vi "Default8bitColourMap.vi"() -> (0 "Default 8-bit Colour Map":u32[](array[numeric]))   [LabVIEW 2020, in "g_ar_toolkit.image.lvlib"]
uses:
  g_ar_toolkit.image.lvlib
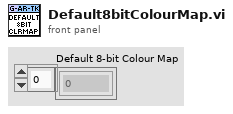
[diagram p1: front panel]
types:
  T1 = cluster{"left":i16, "top":i16, "right":i16, "bottom":i16}
  T2 = typedef "imagedata.ctl" = cluster{"image type":i32, "image depth":i32, "image":u8[], "mask":u8[], "colors":u32[], "Rectangle":cluster{"left":i16, "top":i16, "right":i16, "bottom":i16}}
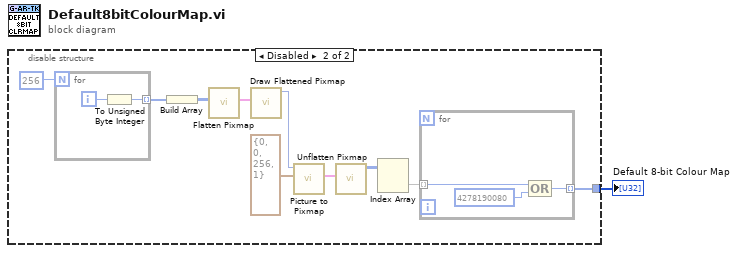
[diagram p0: block diagram]
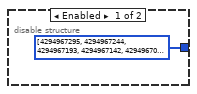
[diagram p2: hidden frame]
diagram:
  n1 = disable-structure shown="Disabled" {
    disable-tunnel: [u32[] [4294967295, 4294967244, 4294967193, 4294967142, 4294967091, 4294967040, 4294954239, 4294954188, 4294954137, 4294954086, 4294954035, 4294953984, 4294941183, 4294941132, 4294941081, 4294941030, 4294940979, 4294940928, 4294928127, 4294928076, 4294928025, 4294927974, 4294927923, 4294927872, 4294915071, 4294915020, 4294914969, 4294914918, 4294914867, 4294914816, 4294902015, 4294901964, 4294901913, 4294901862, 4294901811, 4294901760, 4291624959, 4291624908, 4291624857, 4291624806, 4291624755, 4291624704, 4291611903, 4291611852, 4291611801, 4291611750, 4291611699, 4291611648, 4291598847, 4291598796, 4291598745, 4291598694, 4291598643, 4291598592, 4291585791, 4291585740, 4291585689, 4291585638, 4291585587, 4291585536, 4291572735, 4291572684, 4291572633, 4291572582, 4291572531, 4291572480, 4291559679, 4291559628, 4291559577, 4291559526, 4291559475, 4291559424, 4288282623, 4288282572, 4288282521, 4288282470, 4288282419, 4288282368, 4288269567, 4288269516, 4288269465, 4288269414, 4288269363, 4288269312, 4288256511, 4288256460, 4288256409, 4288256358, 4288256307, 4288256256, 4288243455, 4288243404, 4288243353, 4288243302, 4288243251, 4288243200, 4288230399, 4288230348, 4288230297, 4288230246, 4288230195, 4288230144, 4288217343, 4288217292, 4288217241, 4288217190, 4288217139, 4288217088, 4284940287, 4284940236, 4284940185, 4284940134, 4284940083, 4284940032, 4284927231, 4284927180, 4284927129, 4284927078, 4284927027, 4284926976, 4284914175, 4284914124, 4284914073, 4284914022, 4284913971, 4284913920, 4284901119, 4284901068, 4284901017, 4284900966, 4284900915, 4284900864, 4284888063, 4284888012, 4284887961, 4284887910, 4284887859, 4284887808, 4284875007, 4284874956, 4284874905, 4284874854, 4284874803, 4284874752, 4281597951, 4281597900, 4281597849, 4281597798, 4281597747, 4281597696, 4281584895, 4281584844, 4281584793, 4281584742, 4281584691, 4281584640, 4281571839, 4281571788, 4281571737, 4281571686, 4281571635, 4281571584, 4281558783, 4281558732, 4281558681, 4281558630, 4281558579, 4281558528, 4281545727, 4281545676, 4281545625, 4281545574, 4281545523, 4281545472, 4281532671, 4281532620, 4281532569, 4281532518, 4281532467, 4281532416, 4278255615, 4278255564, 4278255513, 4278255462, 4278255411, 4278255360, 4278242559, 4278242508, 4278242457, 4278242406, 4278242355, 4278242304, 4278229503, 4278229452, 4278229401, 4278229350, 4278229299, 4278229248, 4278216447, 4278216396, 4278216345, 4278216294, 4278216243, 4278216192, 4278203391, 4278203340, 4278203289, 4278203238, 4278203187, 4278203136, 4278190335, 4278190284, 4278190233, 4278190182, 4278190131, 4293787648, 4292673536, 4290445312, 4289331200, 4287102976, 4285988864, 4283760640, 4282646528, 4280418304, 4279304192, 4278251008, 4278246656, 4278237952, 4278233600, 4278224896, 4278220544, 4278211840, 4278207488, 4278198784, 4278194432, 4278190318, 4278190301, 4278190267, 4278190250, 4278190216, 4278190199, 4278190165, 4278190148, 4278190114, 4278190097, 4293848814, 4292730333, 4290493371, 4289374890, 4287137928, 4286019447, 4283782485, 4282664004, 4280427042, 4279308561, 4278190080] ("Array") w3] -> w1
    frame Enabled {
    }
    frame Disabled {
      n2 = for {
        N: 256 -> [_]
        tunnel: [w16] -> w11 mode=indexing
        i -> [w17]
        n3 = To Unsigned Byte Integer(number=w17) -> (unsigned 8bit integer=w16:u8)
      }
      n4 = Build Array(w11) -> (w10:u8[][])
      n5 = call <vilib>:"Flatten Pixmap.vi"("8-bit pixmap"=w10) -> ("image data"=w9:T2)  [unwired: 10 in]
      n6 = call <vilib>:"Draw Flattened Pixmap.vi"("image data"=w9) -> ("new picture"=w8:picture)  [unwired: 8 in]
      n7 = call <vilib>:"Picture to Pixmap.vi"("rect"=T1 {"left"=0, "top"=0, "right"=256, "bottom"=1}, "picture"=w8) -> ("image data"=w6:T2)  [unwired: 8 in, 1 out]
      n8 = call <vilib>:"Unflatten Pixmap.vi"("image data"=w6) -> ("24-bit pixmap"=w5:u32[][])  [unwired: 4 in, 6 out]
      n9 = Index Array(array=w5) -> (element=w4:u32[])  [unwired: 2 in]
      n10 = for {
        tunnel: w4 -> [w15] mode=indexing
        tunnel: [w13] -> w3 mode=indexing
        n11 = Compound Arithmetic op=OR(w15, u32 4278190080 ("value")) -> (w13:u32)
      }
    }
  }
  "Default 8-bit Colour Map" <- w1
